vi "TrigOn.vi"(0 "SystemEvents in":refnum<class "SystemEvents.lvclass">, 1 "event data":T1, 5 "error in (no error)":errorcluster) -> (14 "SystemEvents out":refnum<class "SystemEvents.lvclass">, 19 "error out":errorcluster)   [LabVIEW 2017, in "SystemEvents.lvclass"]
doc: "Fires the TrigOn event with the input parameters in attributes of the event data variant."
uses:
  SystemEvents.lvclass
  SystemEventData/TriggerEventData.ctl
  SystemEvents.lvclass/SystemEvents.ctl
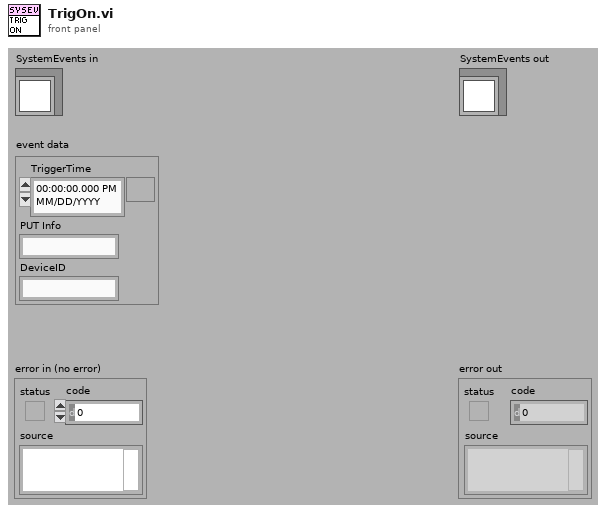
[diagram p1: front panel]
types:
  T1 = typedef "TriggerEventData.ctl" = cluster{"TriggerTime":timestamp, "PUT Info":string, "DeviceID":string}
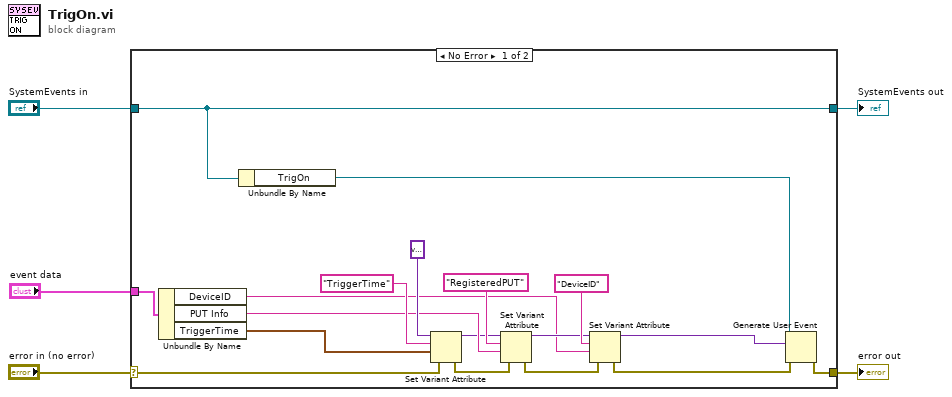
[diagram p0: block diagram]
diagram:
  n1 = case shown="No Error" "error in (no error)" {
    selector: "error in (no error)" -> [w16 w25]
    tunnel: [w22 w25] -> w4
    tunnel: [w23 w24] -> w2
    tunnel: "SystemEvents in" -> [w23 w24]
    tunnel: "event data" -> [w19 _]
    frame No Error {
      n2 = Unbundle By Name(w19) -> ("DeviceID"=w8:string, "PUT Info"=w13:string, "TriggerTime"=w17:timestamp)
      n3 = Unbundle By Name(w23) -> ("TrigOn"=w21:refnum<user-event>)
      n4 = Set Variant Attribute(Variant=variant ("variant"), name="TriggerTime", value=w17, error in=w16) -> (Variant out=w12:variant, error out=w14:errorcluster)  [unwired: 1 out]
      n5 = Set Variant Attribute(Variant=w12, name="RegisteredPUT", value=w13, error in=w14) -> (Variant out=w9:variant, error out=w10:errorcluster)  [unwired: 1 out]
      n6 = Set Variant Attribute(Variant=w9, name="DeviceID", value=w8, error in=w10) -> (Variant out=w6:variant, error out=w7:errorcluster)  [unwired: 1 out]
      n7 = Generate User Event(user event=w21, event data cluster=w6, error in=w7) -> (error out=w22:errorcluster)  [unwired: 1 in, 1 out]
    }
    frame Error {
    }
  }
  "error out" <- w4
  "SystemEvents out" <- w2
